vi "Scale Motor Output.vi"(1 "Exponent":dbl, 2 "Error Input":dbl, 3 "Motor Input":u16) -> (0 "Output":u16)   [LabVIEW 2013, in "ProcessorHelperFunctions.lvlib"]
uses:
  ProcessorHelperFunctions.lvlib
panel:
  # "(0 to 512, 255 = stop)"
  # "Positive number"
  # "(0 to 512, 255 = stop)"
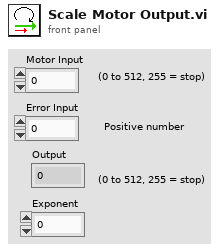
[diagram p1: front panel]
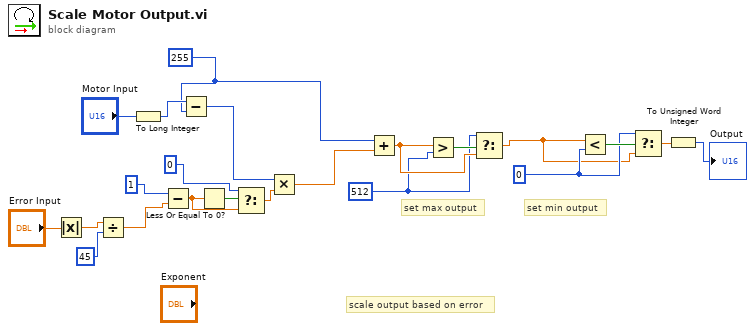
[diagram p0: block diagram]
diagram:
  w12 = 0
  w14 = 512
  w18 = 255
  # "set min output"
  # "set max output"
  # "scale output based on error"
  n1 = Absolute Value(x="Error Input") -> (abs(x)=w7:dbl)
  n2 = Divide(x=w7, y=45) -> (x/y=w8:dbl)
  n3 = To Long Integer(number="Motor Input") -> (32bit integer=w20:i32)
  n4 = Subtract(x=1, y=w8) -> (x-y=w3:dbl)
  n5 = Subtract(x=w20, y=w18) -> (x-y=w19:i32)
  n6 = Less Or Equal To 0?(x=w3) -> (x <= 0?=w4:bool)
  n7 = Select(t=0, s=w4, f=w3) -> (s? t:f=w5:dbl)
  n8 = Multiply(x=w19, y=w5) -> (x*y=w17:dbl)
  n9 = Add(x=w18, y=w17) -> (x+y=w15:dbl)
  n10 = Greater?(x=w15, y=w14) -> (0:w16:bool)
  n11 = Select(t=w14, s=w16, f=w15) -> (s? t:f=w11:dbl)
  n12 = Less?(x=w11, y=w12) -> (x < y?=w13:bool)
  n13 = Select(t=w12, s=w13, f=w11) -> (s? t:f=w10:dbl)
  n14 = To Unsigned Word Integer(number=w10) -> (unsigned 16bit integer=→"Output":u16)
